vi "Datalog to ASCII (DATA, Mode 1).vi"(4 "Error in":errorcluster, 5 "ASCII output path":path=path "C:/Datalogs/Log1_P1.txt", 6 "Precision":i16=4, 7 "Datalog path":path=path "C:/Datalogs/Log1_P1.log") -> (0 "Error out":errorcluster)   [LabVIEW 2015]
uses:
  Ctls/Data values, Mode 1 (for datalog).ctl
  <vilib>/Utility/file.llb/Write Delimited Spreadsheet (string).vi
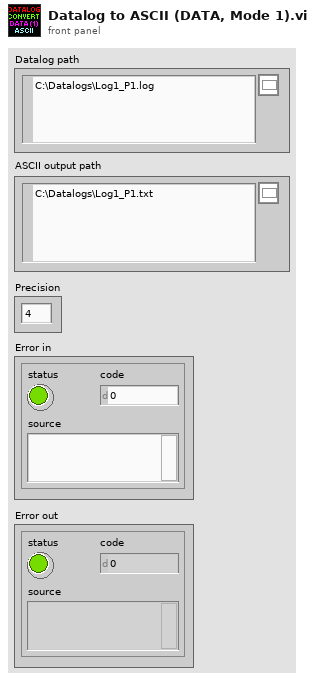
[diagram p1: front panel]
types:
  T1 = typedef "Data values, Mode 1 (for datalog).ctl" = cluster{"Time Stamp":timestamp, "dt (us)":sgl, "dt_warn":u8, "Pressures":sgl[], "Die temps.":sgl[], "Statuses":u8[]}
  T2 = enum16{"open", "replace", "create", "open or create", "replace or create", "replace or create with confirmation"}
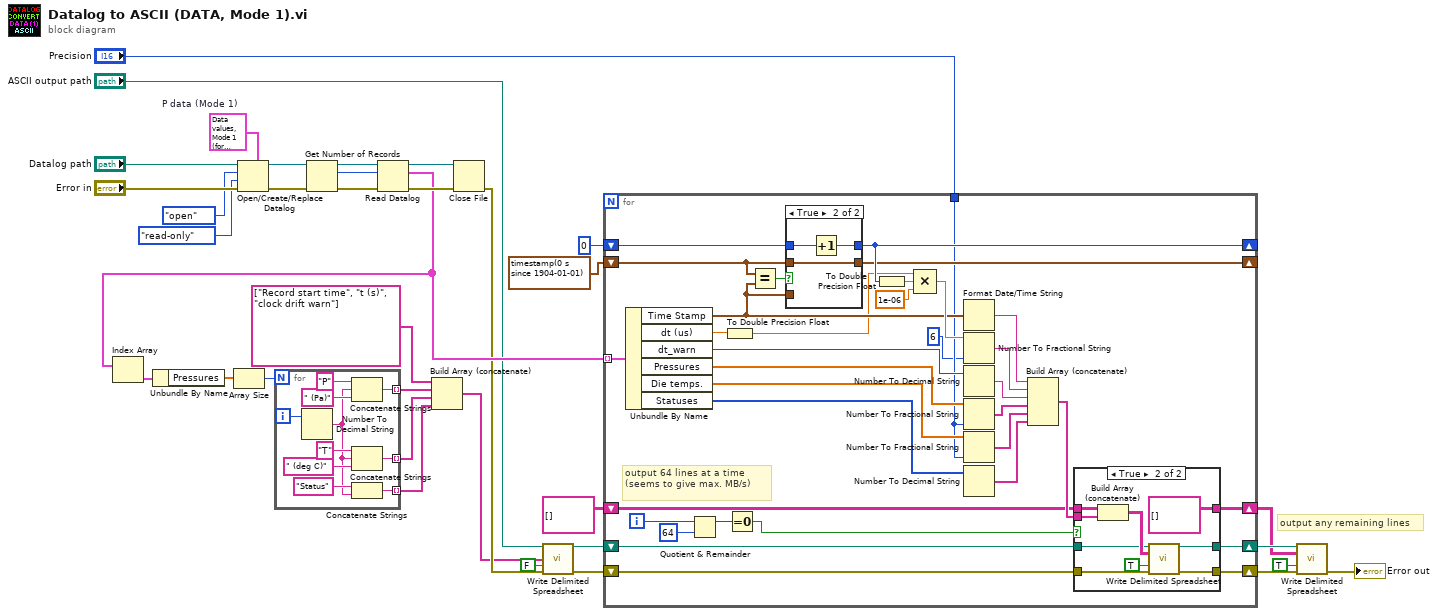
[diagram p0: block diagram]
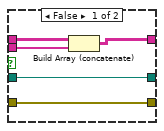
[diagram p2: hidden frame]
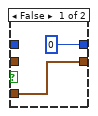
[diagram p3: hidden frame]
diagram:
  w22 = T1 {"Time Stamp"=timestamp(0 s since 1904-01-01), "dt (us)"=0.0, "dt_warn"=0, "Pressures"=[], "Die temps."=[], "Statuses"=[]}  # P data (Mode 1)
  # "output any remaining lines"
  n1 = Open/Create/Replace Datalog(5:w22, 8:"Error in", 9:enum16{"read/write", "read-only", "write-only"}."read-only" ("access (0:read/write)"), 10:T2."open" ("operation (0:open)"), 11:"Datalog path") -> (0:w30:errorcluster, 3:w31:refnum<k1>)  [unwired: 1 in, 1 out]
  n2 = Get Number of Records(4:w30, 7:w31) -> (0:w27:errorcluster, 2:w28:i64, 3:w29:refnum<k1>)
  n3 = Read Datalog(4:w27, 6:w28, 7:w29) -> (0:w25:errorcluster, 2:w13:T1[], 3:w26:refnum<k1>)
  n4 = Index Array(array=w13) -> (element=w15:T1)  [unwired: 1 in]
  n5 = Unbundle By Name(w15) -> ("Pressures"=w16:sgl[])
  n6 = Array Size(array=w16) -> (size(s)=w14:i32)
  n7 = for {
    N: w14 -> [_]
    tunnel: [w38] -> w20 mode=indexing
    tunnel: [w37] -> w19 mode=indexing
    tunnel: [w36] -> w18 mode=indexing
    i -> [w45]
    n8 = Number To Decimal String(number=w45) -> (decimal integer string=w39:string)  [unwired: 1 in]
    n9 = Concatenate Strings("P", w39, " (Pa)") -> (w38:string)
    n10 = Concatenate Strings("T", w39, " (deg C)") -> (w37:string)
    n11 = Concatenate Strings("Status", w39) -> (w36:string)
  }
  n12 = Build Array (concatenate)(string[] ["Record start time", "t (s)", "clock drift warn"], w20, w19, w18) -> (w2:string[])
  n13 = Close File(refnum=w26, error in=w25) -> (error out=w5:errorcluster)  [unwired: 1 out]
  n14 = call-poly <vilib>:"Write Delimited Spreadsheet.vi"("file path (dialog if empty)"="ASCII output path", "1D data"=w2, "append to file? (F)"=FALSE, "error in (no error)"=w5) -> ("new file path (Not A Path if cancelled)"=w7:path, "error out"=w6:errorcluster)  [unwired: 10 in]
  n15 = for {
    tunnel: w13 -> [w70] mode=indexing
    shift-right: [w72] -> _
    shift-left: u32 0 -> [w73]
    shift-right: [w71] -> _
    shift-left: timestamp(0 s since 1904-01-01) ("Time stamp") -> [w74]
    tunnel: "Precision" -> [w61]
    shift-right: [w47] -> w10
    shift-left: w7 -> [w51]
    shift-right: [w46] -> w9
    shift-left: w6 -> [w50]
    shift-right: [w52] -> w1
    shift-left: string[][] [] -> [w53]
    i -> [w55]
    # "output 64 lines at a time (seems to give max. MB/s)"
    n16 = Unbundle By Name(w70) -> ("Time Stamp"=w69:timestamp, "dt (us)"=w68:sgl, "dt_warn"=w66:u8, "Pressures"=w64:sgl[], "Die temps."=w63:sgl[], "Statuses"=w62:u8[])
    n17 = Quotient & Remainder(x=w55, y=64) -> (x-y*floor(x/y)=w56:i32)  [unwired: 1 out]
    n18 = To Double Precision Float(number=w68) -> (double precision float=w67:dbl)
    n19 = Equal To 0?(x=w56) -> (x = 0?=w49:bool)
    n20 = Equal?(x=w74, y=w69) -> (x = y?=w75:bool)
    n21 = case shown="True" w75 {
      tunnel: [u32 0 w98] -> w72
      tunnel: w73 -> [_ w97]
      tunnel: w69 -> [w96 _]
      tunnel: w74 -> [_ w99]
      tunnel: [w96 w99] -> w71
      frame False {
      }
      frame True {
        n22 = Increment(x=w97) -> (x+1=w98:u32)
      }
    }
    n23 = To Double Precision Float(number=w72) -> (double precision float=w80:dbl)
    n24 = Compound Arithmetic op=MULTIPLY(w67, w80, 1e-06 ("value")) -> (w78:dbl)
    n25 = Format Date/Time String(seconds (now)=w69) -> (date/time string=w79:string)  [unwired: 2 in]
    n26 = Number To Fractional String(number=w78, precision (6)=i16 6) -> (F-format string=w77:string)  [unwired: 2 in]
    n27 = Number To Decimal String(number=w66) -> (decimal integer string=w65:string)  [unwired: 1 in]
    n28 = Number To Fractional String(number=w64, precision (6)=w61) -> (F-format string=w60:string[])  [unwired: 2 in]
    n29 = Number To Fractional String(number=w63, precision (6)=w61) -> (F-format string=w59:string[])  [unwired: 2 in]
    n30 = Number To Decimal String(number=w62) -> (decimal integer string=w58:string[])  [unwired: 1 in]
    n31 = Build Array (concatenate)(w79, w77, w65, w60, w59, w58) -> (w54:string[])
    n32 = case shown="True" w49 {
      tunnel: [w85 string[][] []] -> w52
      tunnel: [w82 w93] -> w47
      tunnel: [w81 w92] -> w46
      tunnel: w54 -> [w83 w89]
      tunnel: w53 -> [w84 w88]
      tunnel: w51 -> [w82 w87]
      tunnel: w50 -> [w81 w86]
      frame False {
        n33 = Build Array (concatenate)(w84, w83) -> (w85:string[][])
      }
      frame True {
        n34 = Build Array (concatenate)(w88, w89) -> (w90:string[][])
        n35 = call-poly <vilib>:"Write Delimited Spreadsheet.vi"("file path (dialog if empty)"=w87, "2D data"=w90, "append to file? (F)"=TRUE, "error in (no error)"=w86) -> ("new file path (Not A Path if cancelled)"=w93:path, "error out"=w92:errorcluster)  [unwired: 10 in]
      }
    }
  }
  n36 = call-poly <vilib>:"Write Delimited Spreadsheet.vi"("file path (dialog if empty)"=w10, "2D data"=w1, "append to file? (F)"=TRUE, "error in (no error)"=w9) -> ("error out"=→"Error out":errorcluster)  [unwired: 10 in, 1 out]
